vi "Control Experiment FGV.vi"(6 "Function":enum16{"read", "write"}(ring), 8 "error in (no error)":errorcluster, 11 "Control Experiment.lvclass":refnum<class "Control Experiment.lvclass">) -> (0 "error out":errorcluster, 1 "Unresolved on load":string[](array[string]), 2 "Loaded?":bool, 3 "Control Experiment.lvclass out":refnum<class "Control Experiment.lvclass">)   [LabVIEW 2019, in "Control Experiment.lvclass"]
uses:
  Control Experiment.lvclass
  <vilib>/Utility/sysdir.llb/System Directory Type.ctl
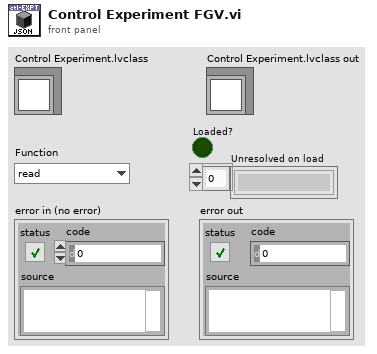
[diagram p1: front panel]
types:
  T1 = typedef "System Directory Type.ctl" = i32
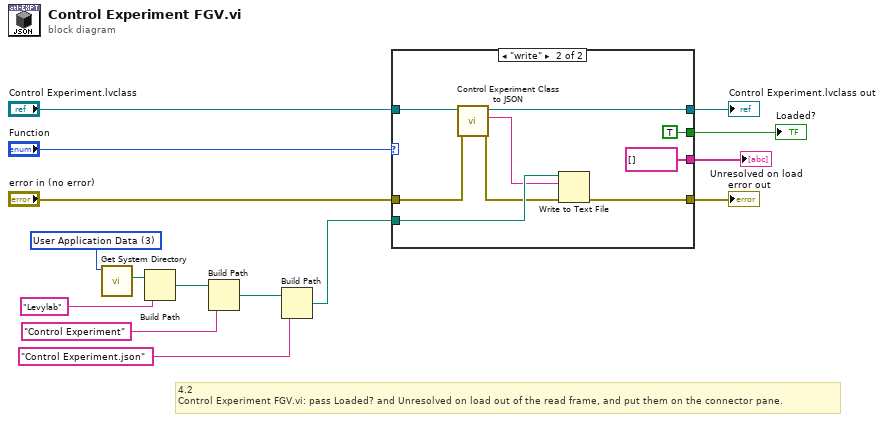
[diagram p0: block diagram]
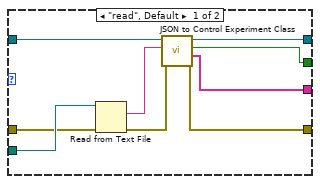
[diagram p2: hidden frame]
diagram:
  w10 = T1 3 items=["User Home"=0, "User Desktop"=1, "User Documents"=2, "User Application Data"=3, "User Preferences"=4, "User Temporary"=5, "Public Documents"=6, "Public Application Data"=7, "Public Preferences"=8, "Public Cache"=13, "System Core Libraries"=9, "System Installed Libraries"=10, "Application Files"=11, "Boot Volume Root"=12] ("system directory type")
  # "4.2\nControl Experiment FGV.vi: pass Loaded? and Unresolved on load out of the read frame, and put them on the connector pane."
  n1 = call <vilib>:"Get System Directory.vi"("system directory type"=w10) -> ("system directory"=w7:path)  [unwired: 10 in]
  n2 = Build Path(base path=w7, name or relative path="Levylab") -> (appended path=w9:path)
  n3 = Build Path(base path=w9, name or relative path="Control Experiment") -> (appended path=w4:path)
  n4 = Build Path(base path=w4, name or relative path="Control Experiment.json") -> (appended path=w5:path)
  n5 = case shown="\"write\"" "Function" {
    tunnel: "Control Experiment.lvclass" -> [w22 w29]
    tunnel: [w18 w30] -> w3
    tunnel: "error in (no error)" -> [w21 w28]
    tunnel: [w19 w32] -> w15
    tunnel: w5 -> [w24 w33]
    tunnel: [w17 string[] [] ("Unresolved on load")] -> w2
    tunnel: [w16 TRUE ("Loaded?")] -> w1
    frame "read", Default {
      n6 = Read from Text File(file (use dialog)=w24, error in=w21) -> (text=w23:string, error out=w20:errorcluster)  [unwired: 2 in, 2 out]
      n7 = call "JSON to Control Experiment Class.vi"("error in (no error)"=w20, "JSON"=w23, "Control Experiment in"=w22) -> ("error out"=w19:errorcluster, "Unresolved on load"=w17:string[], "Loaded?"=w16:bool, "Control Experiment out"=w18:refnum<class "Control Experiment.lvclass">)  [unwired: 5 in]
    }
    frame "write" {
      n8 = call "Control Experiment Class to JSON.vi"("error in (no error)"=w28, "Control Experiment in"=w29) -> ("error out"=w27:errorcluster, "<JSON>"=w31:string, "Control Experiment out"=w30:refnum<class "Control Experiment.lvclass">)  [unwired: 7 in]
      n9 = Write to Text File(file (use dialog)=w33, text=w31, error in=w27) -> (error out=w32:errorcluster)  [unwired: 1 in, 2 out]
    }
  }
  "error out" <- w15
  "Control Experiment.lvclass out" <- w3
  "Unresolved on load" <- w2
  "Loaded?" <- w1
